vi "Word_Get_Range.vi"(4 "end":i32, 6 "start":i32, 8 "error in":errorcluster, 9 "bookmark name":string, 10 "insertion point":u16(ring)=1 items=["begining of document", "end of document", "bookmark", "Custom"], 11 "document in":refnum<k7>) -> (0 "error out (no error)":errorcluster, 1 "range":refnum<k7>, 3 "document out":refnum<k7>)   [LabVIEW 2020, in "NI_ReportGenerationToolkit.lvlib"]
uses:
  <vilib>/addons/_office/NI_ReportGenerationToolkit.lvlib
  <vilib>/Utility/NIReport.llb/NI_ReportGenerationCore.lvlib
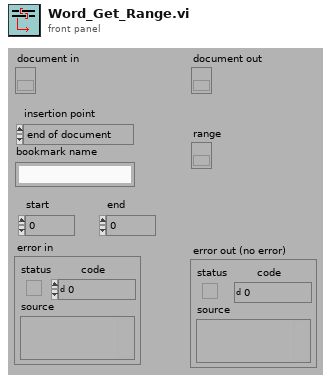
[diagram p1: front panel]
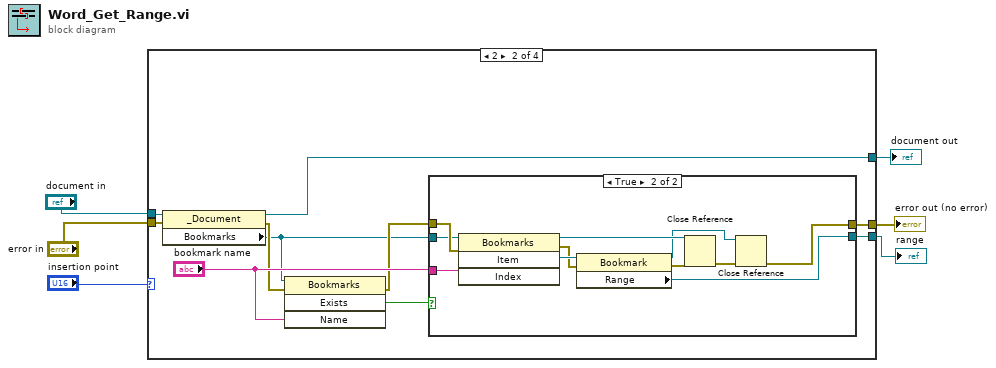
[diagram p0: block diagram]
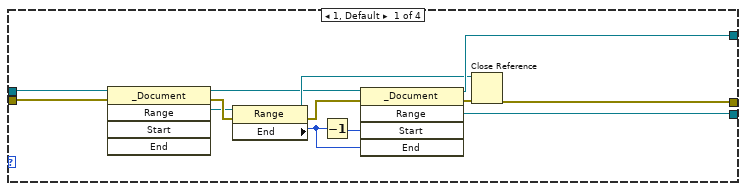
[diagram p2: hidden frame]
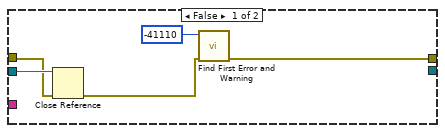
[diagram p3: hidden frame]
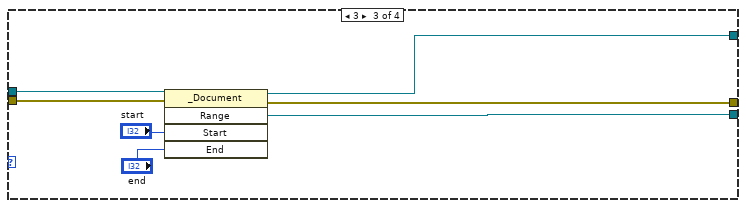
[diagram p4: hidden frame]
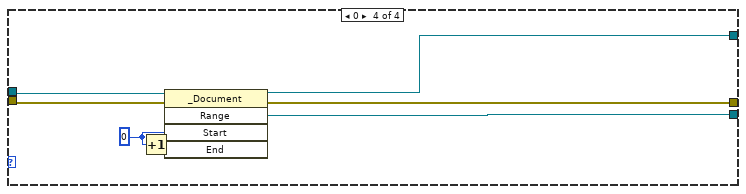
[diagram p5: hidden frame]
diagram:
  n1 = case shown="2" "insertion point" {
    tunnel: [w19 w24 w49 w57] -> w4
    tunnel: "error in" -> [w9 w26 w51 w58]
    tunnel: [w17 w27 w50 w59] -> w1
    tunnel: "document in" -> [w8 w25 w52 w56]
    tunnel: [w7 w23 w46 w53] -> w2
    frame 1, Default {
      n2 = invoke class="_Document" method="Range"(reference=w8, error in=w9) -> (reference out=w13:refnum<k7>, error out=w14:errorcluster, "Range"=w12:refnum<k7>)  [unwired: 3 in, 2 out]
      n3 = property class="Range"(reference=w12, error in=w14) -> (reference out=w15:refnum<k7>, error out=w18:errorcluster, "End"=w11:i32)
      n4 = Decrement(x=w11) -> (x-1=w10:i32)
      n5 = invoke class="_Document" method="Range"(reference=w13, error in=w18, "Start"=w10, "End"=w11) -> (reference out=w19:refnum<k7>, error out=w16:errorcluster, "Range"=w17:refnum<k7>)  [unwired: 1 in, 2 out]
      n6 = Close Reference(reference=w15, error in (no error)=w16) -> (error out=w7:errorcluster)
    }
    frame 2 {
      n7 = property class="_Document"(reference=w25, error in=w26) -> (reference out=w24:refnum<k7>, error out=w22:errorcluster, "Bookmarks"=w20:refnum<k7>)
      n8 = invoke class="Bookmarks" method="Exists"(reference=w20, error in=w22, "Name"="bookmark name") -> (error out=w21:errorcluster, "Exists"=w28:bool)  [unwired: 1 in, 2 out]
      n9 = case shown="True" w28 {
        tunnel: w21 -> [w31 w44]
        tunnel: w20 -> [w32 w38]
        tunnel: "bookmark name" -> [_ w37]
        tunnel: [_ w36] -> w27
        tunnel: [w33 w35] -> w23
        frame False {
          n10 = Close Reference(reference=w32, error in (no error)=w31) -> (error out=w30:errorcluster)
          n11 = call <vilib>:"Find First Error and Warning.vi"("error in (no error)"=w30, "error code"=-41110) -> ("error out"=w33:errorcluster)  [unwired: 5 out]
        }
        frame True {
          n12 = invoke class="Bookmarks" method="Item"(reference=w38, error in=w44, "Index"=w37) -> (reference out=w45:refnum<k7>, error out=w40:errorcluster, "Item"=w43:refnum<k7>)  [unwired: 1 in, 1 out]
          n13 = property class="Bookmark"(reference=w43, error in=w40) -> (reference out=w39:refnum<k7>, error out=w42:errorcluster, "Range"=w36:refnum<k7>)
          n14 = Close Reference(reference=w45, error in (no error)=w42) -> (error out=w41:errorcluster)
          n15 = Close Reference(reference=w39, error in (no error)=w41) -> (error out=w35:errorcluster)
        }
      }
    }
    frame 3 {
      n16 = invoke class="_Document" method="Range"(reference=w52, error in=w51, "Start"="start", "End"="end") -> (reference out=w49:refnum<k7>, error out=w46:errorcluster, "Range"=w50:refnum<k7>)  [unwired: 1 in, 2 out]
    }
    frame 0 {
      w55 = 0
      n17 = Increment(x=w55) -> (x+1=w54:i32)
      n18 = invoke class="_Document" method="Range"(reference=w56, error in=w58, "Start"=w55, "End"=w54) -> (reference out=w57:refnum<k7>, error out=w53:errorcluster, "Range"=w59:refnum<k7>)  [unwired: 1 in, 2 out]
    }
  }
  "range" <- w1
  "error out (no error)" <- w2
  "document out" <- w4
